vi "select_camera.vi"(8 "Camera Error In":errorcluster, 10 "Chosen Camera:":T2, 11 "Camera Session In":T1) -> (0 "Camera Error Out":errorcluster, 2 "Chosen Camera:":T2, 3 "Camera Session Out":T1="cam0", 4 "Session error":errorcluster={"status"=TRUE, "code"=-1, "source"="No session is open"})   [LabVIEW 2014]
uses:
  <vilib>/userdefined/High Color/IMAQdx.ctl
  <vilib>/vision/driver/IMAQdx.llb/IMAQdx Camera Control Mode.ctl
  <vilib>/vision/driver/NI_Vision_Acquisition_Software.lvlib
  <resource>/objmgr/imaqdx.rc
panel:
  in  "Select a camera:":i32(listbox)
  in  "Cancel Button":bool
  in  "Okay":bool
  # "px"
  # "px"
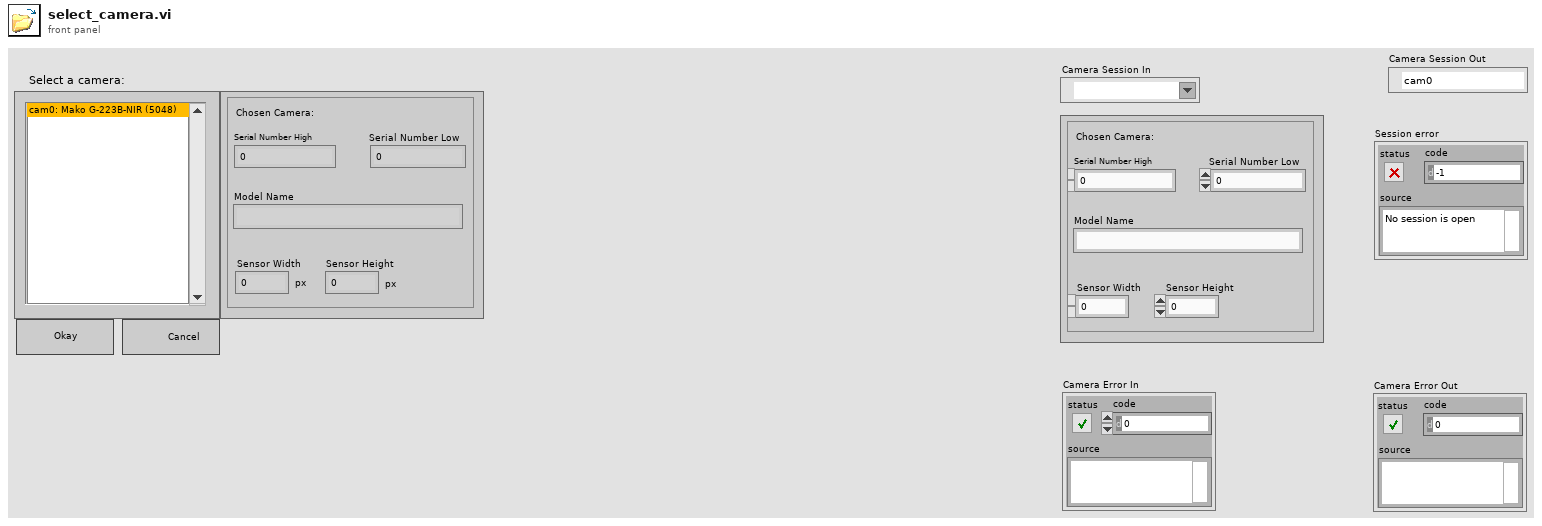
[diagram p1: front panel]
types:
  T1 = typedef "IMAQdx.ctl" = refnum<k21>
  T2 = cluster{"Serial Number High":u32, "Model Name":string, "Sensor Width":u32, "Sensor Height":u32, "Serial Number Low":u32}
  T3 = typedef "NI_Vision_Acquisition_Software.lvlib/IMAQdx Camera Control Mode.ctl" = enum32{"Controller", "Listener"}
  T4 = cluster{"Type":u32, "Version":u32, "Flags":u32, "SerialNumberHigh":u32, "SerialNumberLow":u32, "BusType":u32, "InterfaceName":string, "VendorName":string, "ModelName":string, "CameraFileName":string, "CameraAttributeURL":string}[]
  T5 = cluster{"SerialNumberHigh":u32, "ModelName":string, "Width":u32, "Height":u32, "SerialNumberLow":u32}
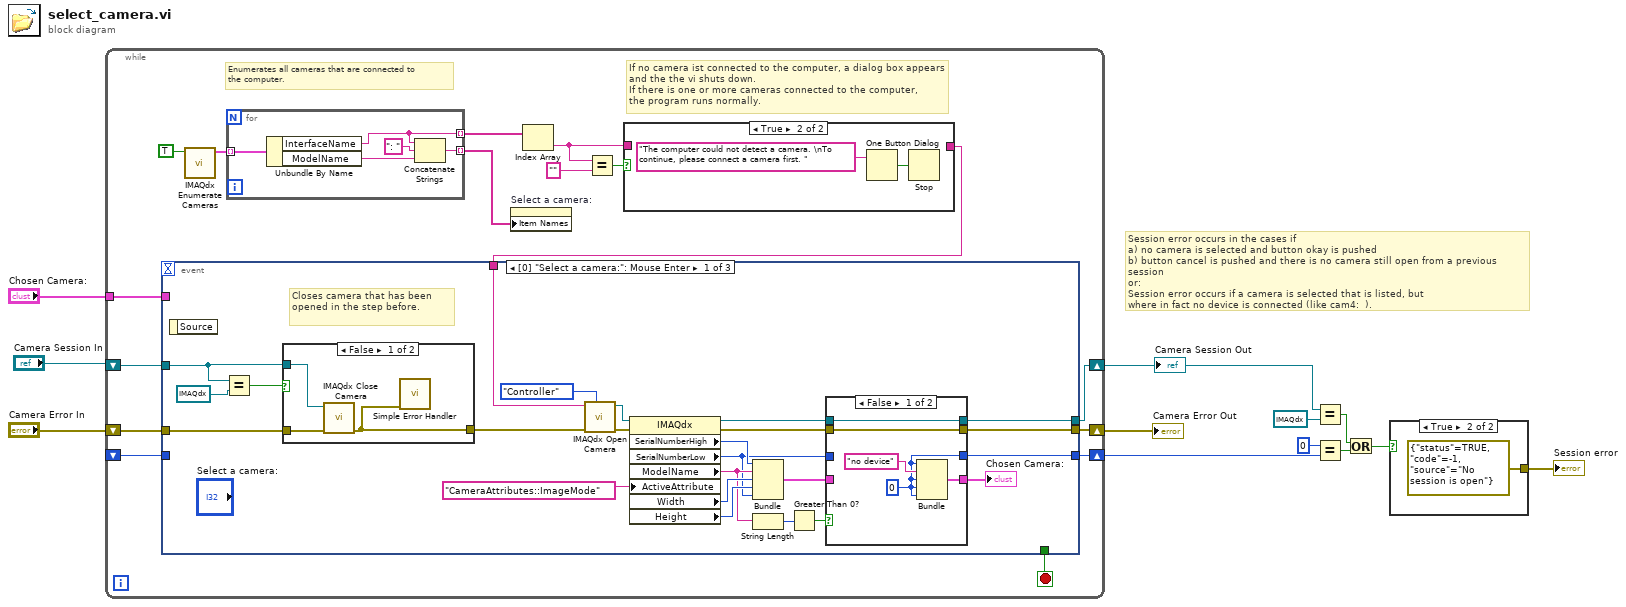
[diagram p0: block diagram]
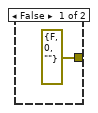
[diagram p2: hidden frame]
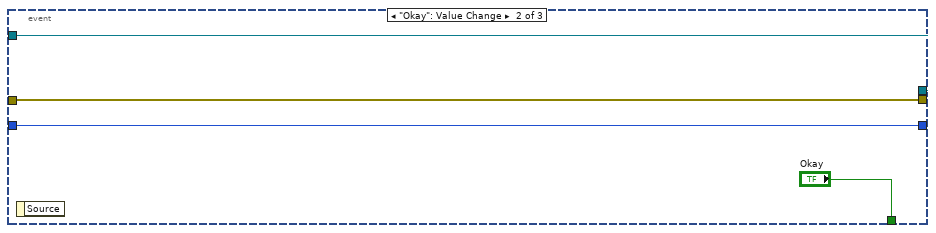
[diagram p6: hidden frame]
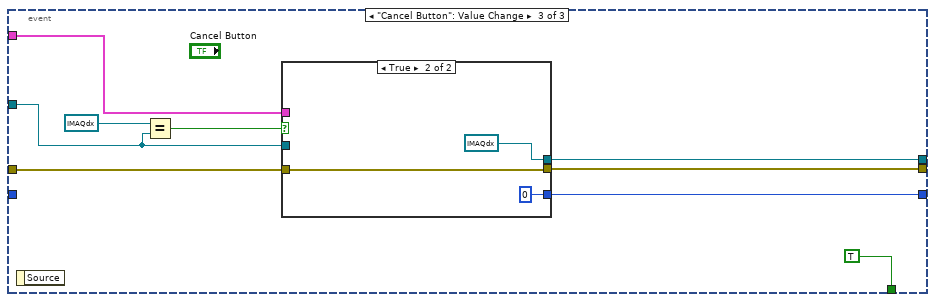
[diagram p7: hidden frame]
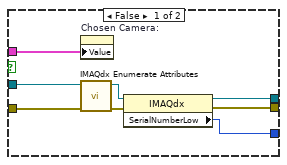
[diagram p8: hidden frame]
diagram:
  # "Session error occurs in the cases if\na) no camera is selected and button okay is pushed\nb) button cancel is pushed and there is no camera still open from a previous session\nor: \nSession error occurs if a camera is selected that is listed, but \nwhere in fact no device is connected (like cam4:  )."
  n1 = while {
    shift-right: [w15] -> w9
    shift-left: "Camera Error In" -> [w25]
    shift-right: [w28] -> w12
    shift-left: "Camera Session In" -> [w27]
    shift-right: [w21] -> w5
    shift-left: _ -> [w20]
    tunnel: "Chosen Camera:" -> [w19]
    stop <- w26 stop-if-true
    # "Enumerates all cameras that are connected to \nthe computer."
    # "If no camera ist connected to the computer, a dialog box appears \nand the the vi shuts down. \nIf there is one or more cameras connected to the computer, \nthe program runs normally."
    n2 = call <vilib>:"IMAQdx Enumerate Cameras.vi"("Connected Only? (Yes)"=TRUE) -> ("Camera Information Array"=w23:T4)  [unwired: 9 in, 1 out]
    n3 = for {
      tunnel: w23 -> [w36] mode=indexing
      tunnel: [w33] -> w22 mode=indexing
      tunnel: [w32] -> w17 mode=indexing
      n4 = Unbundle By Name(w36) -> ("InterfaceName"=w32:string, "ModelName"=w34:string)
      n5 = Concatenate Strings(w32, ": " ("string"), w34) -> (w33:string)
    }
    n6 = property on="Select a camera:" class="LstBox (strict)"("Item Names"=w22) -> ()  [unwired: 2 in, 2 out]
    n7 = Index Array(array=w17) -> (element=w14:string)  [unwired: 1 in]
    n8 = Equal?(x=w14, y="" ("element")) -> (x = y?=w18:bool)
    n9 = case shown="True" w18 {
      tunnel: w14 -> [w29 _]
      tunnel: [w29 _] -> w16
      frame False {
      }
      frame True {
        n10 = One Button Dialog(message="The computer could not detect a camera. \nTo continue, please connect a camera first. ") -> (true=w30:bool)  [unwired: 1 in]
        n11 = Stop(stop? (T)=w30) -> ()
      }
    }
    n12 = event shown="[0] \"Select a camera:\": Mouse Enter" {
      selector: _ -> [_ _ _]
      dyn-events: _ -> [_ _ _]
      timeout: _ -> [_ _ _]
      tunnel: [_ "Okay" TRUE] -> w26
      tunnel: [w60 w76 w84] -> w28
      tunnel: w27 -> [w42 w76 w79]
      tunnel: w25 -> [w40 w74 w81]
      tunnel: w16 -> [w43 _ _]
      tunnel: [w46 w75 w83] -> w21
      tunnel: w20 -> [_ w75 _]
      tunnel: w19 -> [_ _ w82]
      tunnel: [w37 w74 w78] -> w15
      event "Select a camera:": Mouse Enter {
        # "Closes camera that has been opened in the step before."
        n13 = event-data() -> ()  [unwired: 1 in, 1 out]
        n14 = Equal?(x=w42, y=T1 refnum ("Session Out 2")) -> (x = y?=w59:bool)
        n15 = case shown="False" w59 {
          tunnel: w42 -> [w72 _]
          tunnel: w40 -> [w71 w73]
          tunnel: [w70 w73] -> w39
          frame False {
            n16 = call <vilib>:"IMAQdx Close Camera.vi"("error in"=w71, "Session In"=w72) -> ("error out"=w70:errorcluster)  [unwired: 9 in]
            n17 = call <vilib>:"Simple Error Handler.vi"("error in (no error)"=w70) -> ()  [unwired: 4 in, 5 out]
          }
          frame True {
            # "When the program runs the first time, there is no initialised data and no camera that can be closed.  So nothing has to be done."
          }
        }
        n18 = call <vilib>:"IMAQdx Open Camera.vi"("Camera Control Mode"=IMAQdx_Camera_Control_Mode."Controller", "error in"=w39, "Session In"=w43) -> ("error out"=w49:errorcluster, "Session Out"=w50:T1)  [unwired: 7 in]
        n19 = property class="IMAQdx"(reference=w50, error in=w49, "ActiveAttribute"="CameraAttributes::ImageMode") -> (reference out=w51:T1, error out=w38:errorcluster, "SerialNumberHigh"=w58:u32, "SerialNumberLow"=w45:u32, "ModelName"=w52:string, "Width"=w54:u32, "Height"=w53:u32)
        n20 = Bundle("SerialNumberHigh"=w58, "ModelName"=w52, "Width"=w54, "Height"=w53, "SerialNumberLow"=w45) -> (w55:T5)  [unwired: 1 in]
        n21 = String Length(string=w52) -> (length=w57:i32)
        n22 = Greater Than 0?(x=w57) -> (x > 0?=w56:bool)
        n23 = case shown="False" w56 {
          tunnel: [w64 w69] -> w60
          tunnel: w51 -> [w64 w69]
          tunnel: [w62 w68] -> w44
          tunnel: w55 -> [_ w68]
          tunnel: [w63 w67] -> w46
          tunnel: w45 -> [_ w67]
          tunnel: w38 -> [w61 w66]
          tunnel: [w61 w66] -> w37
          frame False {
            w63 = u32 0
            n24 = Bundle(w63, "no device", w63, w63, w63) -> (w62:cluster{u32, string, u32, u32, u32})  [unwired: 1 in]
          }
          frame True {
          }
        }
        "Chosen Camera:" <- w44
      }
      event "Okay": Value Change {
        n25 = event-data() -> ()  [unwired: 1 in, 1 out]
      }
      event "Cancel Button": Value Change {
        n26 = event-data() -> ()  [unwired: 1 in, 1 out]
        n27 = Equal?(x=T1 refnum ("Session Out 2"), y=w79) -> (x = y?=w85:bool)
        n28 = case shown="True" w85 {
          tunnel: [w89 T1 refnum ("Session Out 2")] -> w84
          tunnel: w79 -> [w90 _]
          tunnel: [w92 u32 0 ("SerialNumberLow")] -> w83
          tunnel: [w91 w95] -> w78
          tunnel: w81 -> [w88 w95]
          tunnel: w82 -> [w87 _]
          frame False {
            n29 = property on="Chosen Camera:" class="Clust (strict)"("Value"=w87) -> ()  [unwired: 2 in, 2 out]
            n30 = call <vilib>:"IMAQdx Enumerate Attributes.vi"("error in"=w88, "Session In"=w90) -> ("error out"=w94:errorcluster, "Session Out"=w93:T1)  [unwired: 7 in, 1 out]
            n31 = property class="IMAQdx"(reference=w93, error in=w94) -> (reference out=w89:T1, error out=w91:errorcluster, "SerialNumberLow"=w92:u32)
          }
          frame True {
          }
        }
      }
    }
  }
  "Camera Error Out" <- w9
  "Camera Session Out" <- w12
  n32 = Equal?(x=w12, y=T1 refnum ("Session Out 2")) -> (x = y?=w8:bool)
  n33 = Equal?(x=u32 0, y=w5) -> (x = y?=w6:bool)
  n34 = Or(x=w8, y=w6) -> (x .or. y?=w7:bool)
  n35 = case shown="True" w7 {
    tunnel: [errorcluster {"status"=FALSE, "code"=0, "source"=""} ("error out") errorcluster {"status"=TRUE, "code"=-1, "source"="No session is open"} ("error out")] -> w10
    frame False {
    }
    frame True {
    }
  }
  "Session error" <- w10
